vi "Template to Mask.vi"(7 "order (1.0)":dbl=1.0 min=0.0 format="%.2f", 8 "bandwidth":T1={"bandwidth value"=0.5, "bandwidth unit"=enum."Order"} {"bandwidth value" min=0.0 format="%.2f"}, 9 "window info":T2={"window type"=10, "window length"=2048} {"window type" items=["None"=0, "Hanning"=1, "Hamming"=2, "Blackman-Harris"=3, "Exact Blackman"=4, "Blackman"=5, "Flat Top"=6, "4 Term B-Harris"=7, "7 Term B-Harris"=8, "Low Sidelobe"=9, "Gaussian"=62]; "window length" min=0}, 10 "sampling frequency [S/s]":dbl=1.0 format="%.2f", 11 "Gabor template":dbl[](array[numeric]) format="%.2f") -> (3 "mask array":bool[][](array[boolean]))   [LabVIEW 2017, in "SoundVib_Gabor.lvlib"]
doc: "Creates a binary mask for <B>order</B>."
uses:
  <vilib>/addons/Sound and Vibration/Order Analysis/Gabor Order Tracking/SoundVib_Gabor.lvlib
  <vilib>/addons/Sound and Vibration/Order Analysis/Ref Gabor Order Tracking/window information.ctl
  <vilib>/addons/Sound and Vibration/Order Analysis/Ref Gabor Order Tracking/Mask Bandwidth.ctl
panel:
  # "Template to Mask"
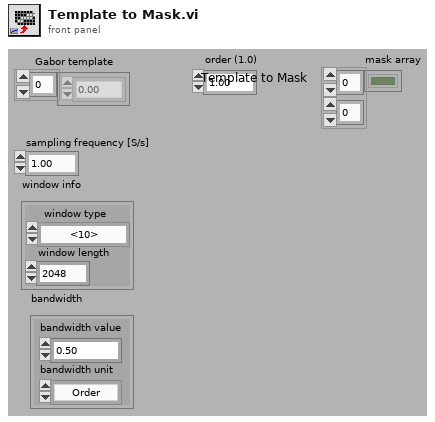
[diagram p1: front panel]
types:
  T1 = typedef "SoundVib_Gabor.lvlib/Mask Bandwidth.ctl" = cluster{"bandwidth value":dbl, "bandwidth unit":enum16{"Order", "Hz"}}
  T2 = typedef "SoundVib_Gabor.lvlib/window information.ctl" = cluster{"window type":u32, "window length":i32}
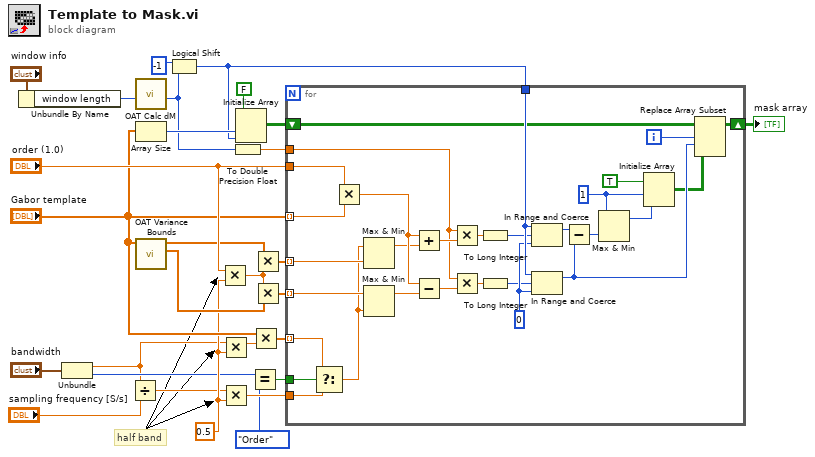
[diagram p0: block diagram]
diagram:
  w10 = 0.5
  # "half band"
  n1 = Unbundle By Name("window info") -> ("window length"=w15:i32)
  n2 = Unbundle("bandwidth") -> ("bandwidth value"=w6:dbl, "bandwidth unit"=w7:enum16{"Order", "Hz"})
  n3 = Divide(x=w6, y="sampling frequency [S/s]") -> (x/y=w4:dbl)
  n4 = call <vilib>:"OAT Calc dM.vi"("window length"=w15) -> ("actual window length"=w14:i32)  [unwired: 7 in, 3 out]
  n5 = Array Size(array="Gabor template") -> (size(s)=w25:i32)
  n6 = call <vilib>:"OAT Variance Bounds.vi"("center frequencies"="Gabor template") -> ("lower bounds"=w19:dbl[], "upper bounds"=w20:dbl[])  [unwired: 9 in]
  n7 = Logical Shift(y=-1, x=w14) -> (x << y=w1:i32)
  n8 = Multiply(x="order (1.0)", y=w10) -> (x*y=w18:dbl)
  n9 = Multiply(x=w6, y=w10) -> (x*y=w12:dbl)
  n10 = Multiply(x=w4, y=w10) -> (x*y=w11:dbl)
  n11 = To Double Precision Float(number=w14) -> (double precision float=w3:dbl)
  n12 = Initialize Array(FALSE, w25, w1) -> (w27:bool[][])
  n13 = Equal?(x=w7, y=enum16{"Order", "Hz"}."Order" ("unit")) -> (x = y?=w16:bool)
  n14 = Multiply(x="Gabor template", y=w12) -> (x*y=w9:dbl[])
  n15 = Multiply(x=w20, y=w18) -> (x*y=w22:dbl[])
  n16 = Multiply(x=w18, y=w19) -> (x*y=w23:dbl[])
  n17 = for {
    shift-right: [w43] -> w2
    shift-left: w27 -> [w44]
    tunnel: w1 -> [w56]
    tunnel: "order (1.0)" -> [w58]
    tunnel: "Gabor template" -> [w57] mode=indexing
    tunnel: w23 -> [w33] mode=indexing
    tunnel: w22 -> [w34] mode=indexing
    tunnel: w3 -> [w46]
    tunnel: w16 -> [w32]
    tunnel: w11 -> [w30]
    tunnel: w9 -> [w29] mode=indexing
    i -> [w42]
    w37 = 1 ("Dimension Size")
    w54 = 0
    n18 = Select(t=w29, s=w32, f=w30) -> (s? t:f=w31:dbl)
    n19 = Multiply(x=w58, y=w57) -> (x*y=w49:dbl)
    n20 = Max & Min(x=w31, y=w34) -> (max(x,y)=w36:dbl)  [unwired: 1 out]
    n21 = Max & Min(x=w33, y=w31) -> (max(x,y)=w35:dbl)  [unwired: 1 out]
    n22 = Add(x=w49, y=w36) -> (x+y=w51:dbl)
    n23 = Subtract(x=w49, y=w35) -> (x-y=w55:dbl)
    n24 = Multiply(x=w46, y=w51) -> (x*y=w48:dbl)
    n25 = Multiply(x=w46, y=w55) -> (x*y=w47:dbl)
    n26 = To Long Integer(number=w48) -> (32bit integer=w50:i32)
    n27 = To Long Integer(number=w47) -> (32bit integer=w53:i32)
    n28 = In Range and Coerce(upper limit=w56, x=w50, lower limit=w54) -> (coerced(x)=w52:i32)  [unwired: 1 out]
    n29 = In Range and Coerce(upper limit=w56, x=w53, lower limit=w54) -> (coerced(x)=w41:i32)  [unwired: 1 out]
    n30 = Subtract(x=w52, y=w41) -> (x-y=w39:i32)
    n31 = Max & Min(x=w37, y=w39) -> (max(x,y)=w38:i32)  [unwired: 1 out]
    n32 = Initialize Array(TRUE, w37, w38) -> (w40:bool[][])
    n33 = Replace Array Subset(array=w44, new element=w40, index (row)=w42, index (col)=w41) -> (w43:bool[][])
  }
  "mask array" <- w2
